vi "ConfigureSimulatedData.vi"() -> (3 "Sim Config Refs":T1)   [LabVIEW 2017, in "ScanEngine.lvlib"]
uses:
  <vilib>/addons/InsightCM/Devices/Shared/Common/ScanEngine/ScanEngine.lvlib
  <vilib>/addons/InsightCM/Devices/Shared/Common/ScanEngine/controls/SimulatedData.ctl
  <vilib>/addons/InsightCM/Devices/Shared/Common/ScanEngine/controls/SimConfigRefs.ctl
  <vilib>/addons/InsightCM/Devices/Shared/Common/ScanEngine/subVIs/SimulatedConfigRefGlobal.vi
  <vilib>/addons/InsightCM/Devices/Shared/Cms/CmsAcquisition/subVIs/SimulatedConfigRefGlobal.vi
  <vilib>/addons/InsightCM/Devices/Shared/Cms/CmsAcquisition/CmsAcquisition.lvlib
panel:
  in  "Sim Config":T2[](array[typedef])
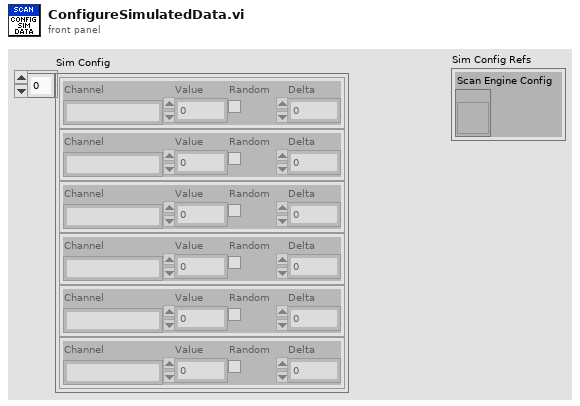
[diagram p1: front panel]
types:
  T1 = typedef "ScanEngine.lvlib/SimConfigRefs.ctl" = cluster{"Scan Engine Config":refnum<vi>}
  T2 = typedef "ScanEngine.lvlib/SimulatedData.ctl" = cluster{"Channel":string, "Value":dbl, "Random":bool, "Delta":dbl}
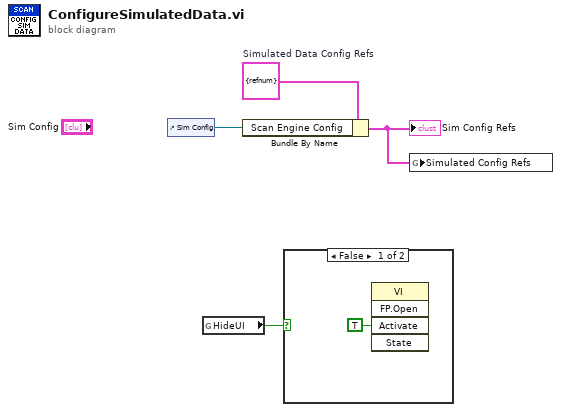
[diagram p0: block diagram]
diagram:
  w4 = T1 {"Scan Engine Config"=refnum}  # Simulated Data Config Refs
  n1 = control-ref of="Sim Config"() -> (w3:refnum<vi>)
  n2 = global read "SimulatedConfigRefGlobal.vi" "HideUI"() -> (w1:bool)
  n3 = Bundle By Name(cluster=w4, "Scan Engine Config"=w3) -> (w2:T1)
  "Sim Config Refs" <- w2
  n4 = case shown="False" w1 {
    frame False {
      n5 = invoke class="VI" method="FP.Open"("Activate"=TRUE ("Activate?")) -> ()  [unwired: 4 in, 5 out]
    }
    frame True {
    }
  }
  n6 = global write "SimulatedConfigRefGlobal.vi" "Simulated Config Refs"(w2) -> ()
